vi "PH_DeformableMirror.ProcEvents.vi"(0 "i ref in":refnum<vi>, 5 "error in":errorcluster) -> (14 "i ref out":refnum<vi>, 19 "error out":errorcluster)   [LabVIEW 2014, in "PH_DeformableMirror.lvlib"]
doc: "This method is used to define the events the object will listen to. Add your own events here."
uses:
  PH_DeformableMirror.lvlib
  CSCore/BaseProcess/BaseProcess.event definition.ctl
  CSCore/CAEObj/CAEObj.event definition.ctl
  CSCore/BaseProcess/BaseProcess.descriptor string definition.ctl
  CSCore/BaseProcess/BaseProcess.lvlib
  CSCore/CAEObj/CAEObj.lvlib
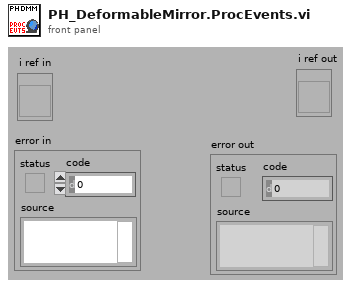
[diagram p1: front panel]
types:
  T1 = typedef "BaseProcess.lvlib/BaseProcess.event definition.ctl" = cluster{"CAEEvtDef":T2, "Data Descriptor":T3}
  T2 = typedef "CAEObj.lvlib/CAEObj.event definition.ctl" = cluster{"URL":string, "enable":bool, "ignoreResID":bool}
  T3 = typedef "BaseProcess.lvlib/BaseProcess.descriptor string definition.ctl" = string
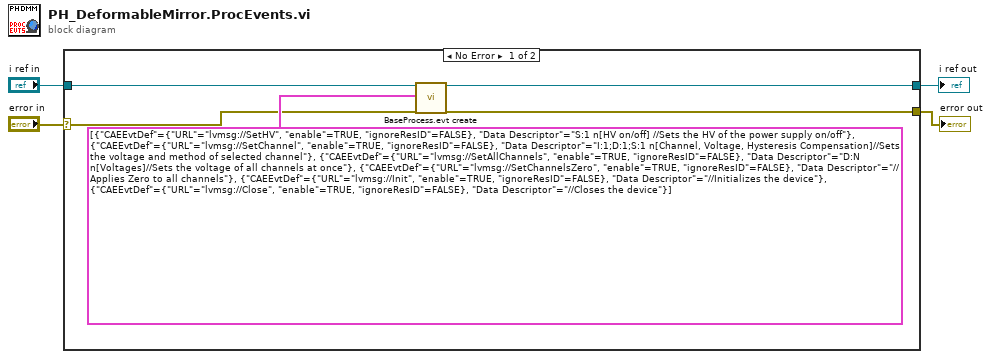
[diagram p0: block diagram]
diagram:
  n1 = case shown="No Error" "error in" {
    selector: "error in" -> [w5 w10]
    tunnel: "i ref in" -> [w9 w11]
    tunnel: [w8 w11] -> w3
    tunnel: [w7 w10] -> w2
    frame No Error {
      n2 = call "BaseProcess.evt create.vi"("i ref in"=w9, "newEvents"=T1[] [{"CAEEvtDef"={"URL"="lvmsg://SetHV", "enable"=TRUE, "ignoreResID"=FALSE}, "Data Descriptor"="S:1 n[HV on/off] //Sets the HV of the power supply on/off"}, {"CAEEvtDef"={"URL"="lvmsg://SetChannel", "enable"=TRUE, "ignoreResID"=FALSE}, "Data Descriptor"="I:1;D:1;S:1 n[Channel, Voltage, Hysteresis Compensation]//Sets the voltage and method of selected channel"}, {"CAEEvtDef"={"URL"="lvmsg://SetAllChannels", "enable"=TRUE, "ignoreResID"=FALSE}, "Data Descriptor"="D:N n[Voltages]//Sets the voltage of all channels at once"}, {"CAEEvtDef"={"URL"="lvmsg://SetChannelsZero", "enable"=TRUE, "ignoreResID"=FALSE}, "Data Descriptor"="//Applies Zero to all channels"}, {"CAEEvtDef"={"URL"="lvmsg://Init", "enable"=TRUE, "ignoreResID"=FALSE}, "Data Descriptor"="//Initializes the device"}, {"CAEEvtDef"={"URL"="lvmsg://Close", "enable"=TRUE, "ignoreResID"=FALSE}, "Data Descriptor"="//Closes the device"}] ("new events"), "error in (no error)"=w5) -> ("i ref out"=w8:refnum<vi>, "error out"=w7:errorcluster)  [unwired: 13 in, 2 out]
    }
    frame Error {
    }
  }
  "i ref out" <- w3
  "error out" <- w2
